vi "myRIO-1900 Customized FPGA.vi"() -> ()   [LabVIEW 2021]
doc: "This VI contains the default FPGA personality in addition to code that generates a sine waveform and filtered sine waveform based on parameters set by RT Main.vi. Keeping the default personality allows you to continue using the myRIO APIs even after adding custom FPGA code."
uses:
  <vilib>/eio/EIONode/EIONode.xnode
  <vilib>/rvi/eio/common/nirviEmuTemplateMethod_errors.vi
  <vilib>/Platform/TimedLoop/XDataNode/wakeup.ctl
  <vilib>/Platform/TimedLoop/XDataNode/XDNodeRunTimeDep.lvlib
  <vilib>/Platform/TimedLoop/XDataNode/nitl_modes.ctl
  <vilib>/Platform/TimedLoop/XDataNode/timing_clust.ctl
  <vilib>/Platform/TimedLoop/XDataNode/XDataNode.xnode
  <vilib>/rvi/Analysis/measure/notch/XNode/niFpgaNotchFilter.xnode
  <vilib>/rvi/DataTransferAndStorage/Container/XNode/niFpgaContainer.xnode
  <vilib>/rvi/interface/RandomDataEmulation/nirviRandomDataFpgaReadWriteTemplate.vi
  <vilib>/rvi/LocalResourceManager/LocalResourceManager.xnode
  <vilib>/rvi/eio/common/nirviEmuReportErrorAndStop.vi
  <vilib>/rvi/DataTransferAndStorage/Container/Common/niFpgaContainerGetUniqueNameForEmu.vi
  <vilib>/rvi/DataTransferAndStorage/Container/Common/niFpgaContainerSetEmuInfo.vi
  <vilib>/rvi/FIFO/Fifo_Resource/nirvififoEmulationRead.vi
  <vilib>/rvi/FIFO/Fifo_Resource/nirvififoEmulationWrite.vi
  Sub VIs/Utilities/Start Boolean.ctl
panel:
  in  "SPI.A.IRQ.NO":u8=15
  in  "SPI.B.IRQ.NO":u8=15
  out "ACC.Z.VAL 2":u16
  out "SYS.ACC.RDY":bool
  out "ACC.Y.VAL 2":u16
  out "ACC.X.VAL 2":u16
  in  "Stop":bool
  in  "Sine wave properties":T1={"Frequency (periods/tick)"=0.0002500000409781933, "Phase offset (periods)"=0.0, "Scale factor"=1.0, "Amplitude offset"=0.0}
  in  "Initialize":bool
  in  "Filter scaled coefficients":i32[](array[numeric])=[-917062152, 995401988, -1407710991]
  out "Actual loop rate":u32=1000
  in  "Desired loop rate (ticks)":u32=1000
  out "AO.SYS.STAT":bool
  out "DI.BTN":u8 format="%08b"
  in  "DO.LED3:0":u8 format="%04b"
  in  "AO.SYS.GO":T2
  in  "AO.AudioOut_L.VAL":u16
  in  "AO.AudioOut_R.VAL":u16
  out "AI.AudioIn_L.VAL":u16
  out "AI.AudioIn_R.VAL":u16
  in  "DIO.B_15:8.OUT":u8 format="%08b"
  in  "DIO.B_15:8.DIR":u8 format="%08b"
  out "DIO.B_15:8.IN":u8 format="%08b"
  in  "DIO.A_15:8.DIR":u8 format="%08b"
  in  "DIO.A_15:8.OUT":u8 format="%08b"
  out "DIO.A_15:8.IN":u8 format="%08b"
  in  "PWM.C_0.MAX":u16
  in  "PWM.C_0.CMP":u16
  out "PWM.C_0.CNTR":u16
  in  "PWM.C_0.CNFG":u8 format="%08b"
  in  "PWM.C_0.CS":u8
  in  "PWM.C_1.MAX":u16
  in  "PWM.C_1.CMP":u16
  out "PWM.C_1.CNTR":u16
  in  "PWM.C_1.CNFG":u8 format="%08b"
  in  "PWM.C_1.CS":u8
  out "ENC.C_1.STAT":u8 format="%08b"
  out "ENC.C_1.CNTR":u32
  in  "ENC.C_1.CNFG":u8 format="%08b"
  out "ENC.C_0.STAT":u8 format="%08b"
  out "ENC.C_0.CNTR":u32
  in  "ENC.C_0.CNFG":u8 format="%08b"
  in  "SYS.SELECTA":u8 format="%08b"
  in  "SYS.SELECTC":u8 format="%08b"
  in  "SYS.SELECTB":u8 format="%08b"
  in  "AO.C_1.VAL":u16
  in  "AO.C_0.VAL":u16
  out "AI.C_0.VAL":u16
  out "AI.C_1.VAL":u16
  in  "DIO.C_7:0.OUT":u8 format="%08b"
  in  "DIO.C_7:0.DIR":u8 format="%08b"
  out "DIO.C_7:0.IN":u8 format="%08b"
  in  "DIO.A_7:0.DIR":u8 format="%08b"
  in  "DIO.A_7:0.OUT":u8 format="%08b"
  out "DIO.A_7:0.IN":u8 format="%08b"
  in  "PWM.B_0.CMP":u16
  in  "PWM.B_0.MAX":u16
  out "PWM.B_0.CNTR":u16
  in  "PWM.B_0.CNFG":u8 format="%08b"
  in  "PWM.B_0.CS":u8
  in  "PWM.B_1.CMP":u16
  in  "PWM.B_1.MAX":u16
  out "PWM.B_1.CNTR":u16
  in  "PWM.B_1.CNFG":u8 format="%08b"
  in  "PWM.B_1.CS":u8
  in  "PWM.B_2.CMP":u16
  in  "PWM.B_2.MAX":u16
  out "PWM.B_2.CNTR":u16
  in  "PWM.B_2.CNFG":u8 format="%08b"
  in  "PWM.B_2.CS":u8
  out "SYS.RDY":bool
  out "SYS.AI.RDY":bool
  in  "I2C.B.GO":T2
  in  "I2C.A.GO":T2
  in  "I2C.A.CNFG":u8 format="%08b"
  in  "I2C.B.CNFG":u8 format="%08b"
  in  "I2C.A.DATO":u8
  out "I2C.A.DATI":u8
  in  "I2C.A.ADDR":u8 format="%08b"
  in  "I2C.A.CNTR":u8
  in  "I2C.B.DATO":u8
  out "I2C.B.DATI":u8
  in  "I2C.B.ADDR":u8 format="%08.0f"
  in  "I2C.B.CNTR":u8
  in  "I2C.A.CNTL":u8 format="%08b"
  out "I2C.A.STAT":u8 format="%08b"
  in  "I2C.B.CNTL":u8 format="%08b"
  out "I2C.B.STAT":u8 format="%08b"
  out "SPI.B.STAT":u8 format="%08b"
  in  "SPI.B.GO":T2
  out "SPI.A.STAT":u8 format="%08b"
  in  "SPI.A.GO":T2
  out "ENC.B.STAT":u8 format="%08b"
  out "ENC.A.STAT":u8 format="%08b"
  out "ENC.B.CNTR":u32
  out "ENC.A.CNTR":u32
  in  "ENC.B.CNFG":u8 format="%08b"
  in  "ENC.A.CNFG":u8 format="%08b"
  in  "SPI.B.DATO":u16
  out "SPI.B.DATI":u16
  in  "SPI.B.CNFG":u16 format="%016.0f"
  in  "SPI.B.CNT":u16
  in  "SPI.A.CNT":u16
  in  "SPI.A.CNFG":u16 format="%016b"
  out "SPI.A.DATI":u16
  in  "SPI.A.DATO":u16
  in  "PWM.A_0.MAX":u16
  in  "PWM.A_0.CMP":u16
  out "PWM.A_0.CNTR":u16
  in  "PWM.A_0.CNFG":u8 format="%08b"
  in  "PWM.A_0.CS":u8
  in  "PWM.A_1.CMP":u16
  in  "PWM.A_1.MAX":u16
  out "PWM.A_1.CNTR":u16
  in  "PWM.A_1.CNFG":u8 format="%08b"
  in  "PWM.A_1.CS":u8
  in  "PWM.A_2.CMP":u16
  in  "PWM.A_2.MAX":u16
  out "PWM.A_2.CNTR":u16
  in  "PWM.A_2.CNFG":u8 format="%08b"
  in  "PWM.A_2.CS":u8
  in  "DIO.B_7:0.OUT":u8 format="%08b"
  in  "DIO.B_7:0.DIR":u8 format="%08b"
  out "DIO.B_7:0.IN":u8 format="%08b"
  out "AI.A_0.VAL":u16
  out "AI.A_1.VAL":u16
  out "AI.A_2.VAL":u16
  out "AI.A_3.VAL":u16
  out "AI.B_0.VAL":u16
  out "AI.B_1.VAL":u16
  out "AI.B_2.VAL":u16
  out "AI.B_3.VAL":u16
  in  "AO.B_1.VAL":u16
  in  "AO.B_0.VAL":u16
  in  "AO.A_1.VAL":u16
  in  "AO.A_0.VAL":u16
  # "System"
  # "Onboard Devices"
  # "Connector A"
  # "Connector B"
  # "Connector C"
  # "Audio Connector"
  # "Accelerometer"
  # "Analog Input"
  # "Analog Output"
  # "Digital I/O"
  # "Counters / PWM"
  # "SPI Master"
  # "Analog Input"
  # "Analog Output"
  # "Digital I/O"
  # "Counters / PWM"
  # "SPI Master"
  # "Analog Input"
  # "Analog Output"
  # "Digital I/O"
  # "Counters / PWM"
  # "Analog Input"
  # "Analog Output"
  # "Encoders"
  # "IO Configuration"
  # "Buttons & LEDs"
  # "IO Configuration"
  # "IO Configuration"
  # "Encoders"
  # "Encoders"
  # "I2C Master"
  # "I2C Master"
  # "This VI contains the default FPGA personality in addition to code that generates a sine waveform and filtered sine waveform based on parameters set by RT Main.vi. Keeping the default personality allows you to continue using the myRIO APIs even after adding custom FPGA code."
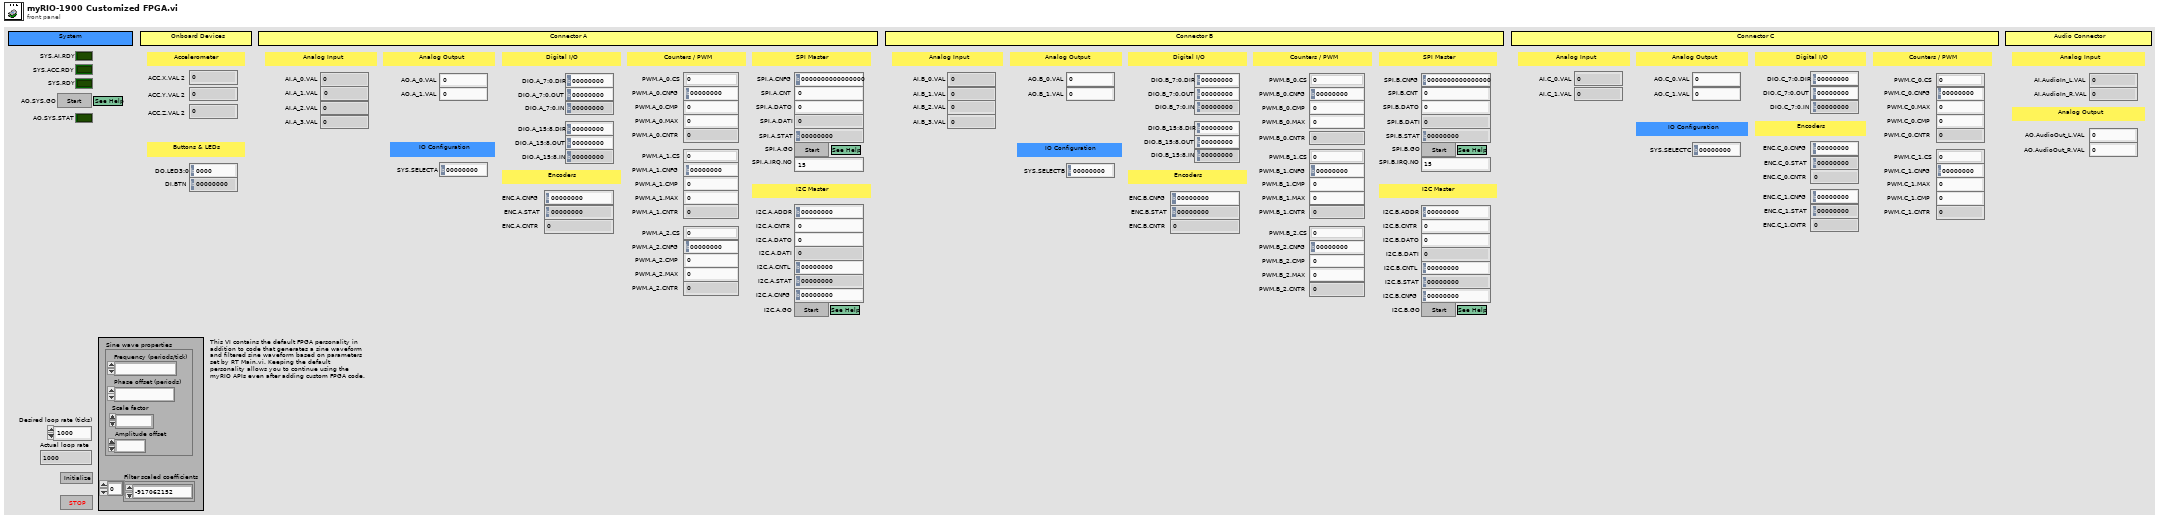
[diagram p1: front panel]
types:
  T1 = cluster{"Frequency (periods/tick)":fxp<+,32,0>, "Phase offset (periods)":fxp<+,32,0>, "Scale factor":fxp<+,12,1>, "Amplitude offset":fxp<+/-,16,12>}
  T2 = typedef "Start Boolean.ctl" = bool
  T3 = typedef "XDNodeRunTimeDep.lvlib/timing_clust.ctl" = cluster{"Expected End [f-1]":u64, "Actual End [f-1]":u64, "Finished Late? [f-1]":bool, "Expected End [i-1]":u64, "Actual End [i-1]":u64, "Finished Late? [i-1]":bool, "Expected Start [i]":u64, "Actual Start [i]":u64, "Expected Start [f]":u64, "Actual Start [f]":u64, "Source Name":string, "Structure Name":string, "Period":i64, "Deadline":i64, "Offset":i64, "Start":i64, "Priority":i32, "Timeout":i32, "Mode":T4, "Wakeup Reason":T5, "Error":errorcluster, "Source Type":string, "Secondary Source Type":string, "Global End Time":u64, "Global Start Time":u64, "Frame Duration":u64, "Iteration Duration":u64, "Assigned CPU":i32, "I/O Scan Engine Mode":u32}
  T4 = typedef "XDNodeRunTimeDep.lvlib/nitl_modes.ctl" = enum32{"No Change", "Process missed periods, maintain original phase", "Discard missed periods, maintain original phase", "Process missed periods, ignore original phase", "Discard missed periods, ignore original phase"}
  T5 = typedef "XDNodeRunTimeDep.lvlib/wakeup.ctl" = enum32{"Normal", "Aborted", "Asynchronous wakeup", "Timing source error", "Timed loop error", "Timeout"}
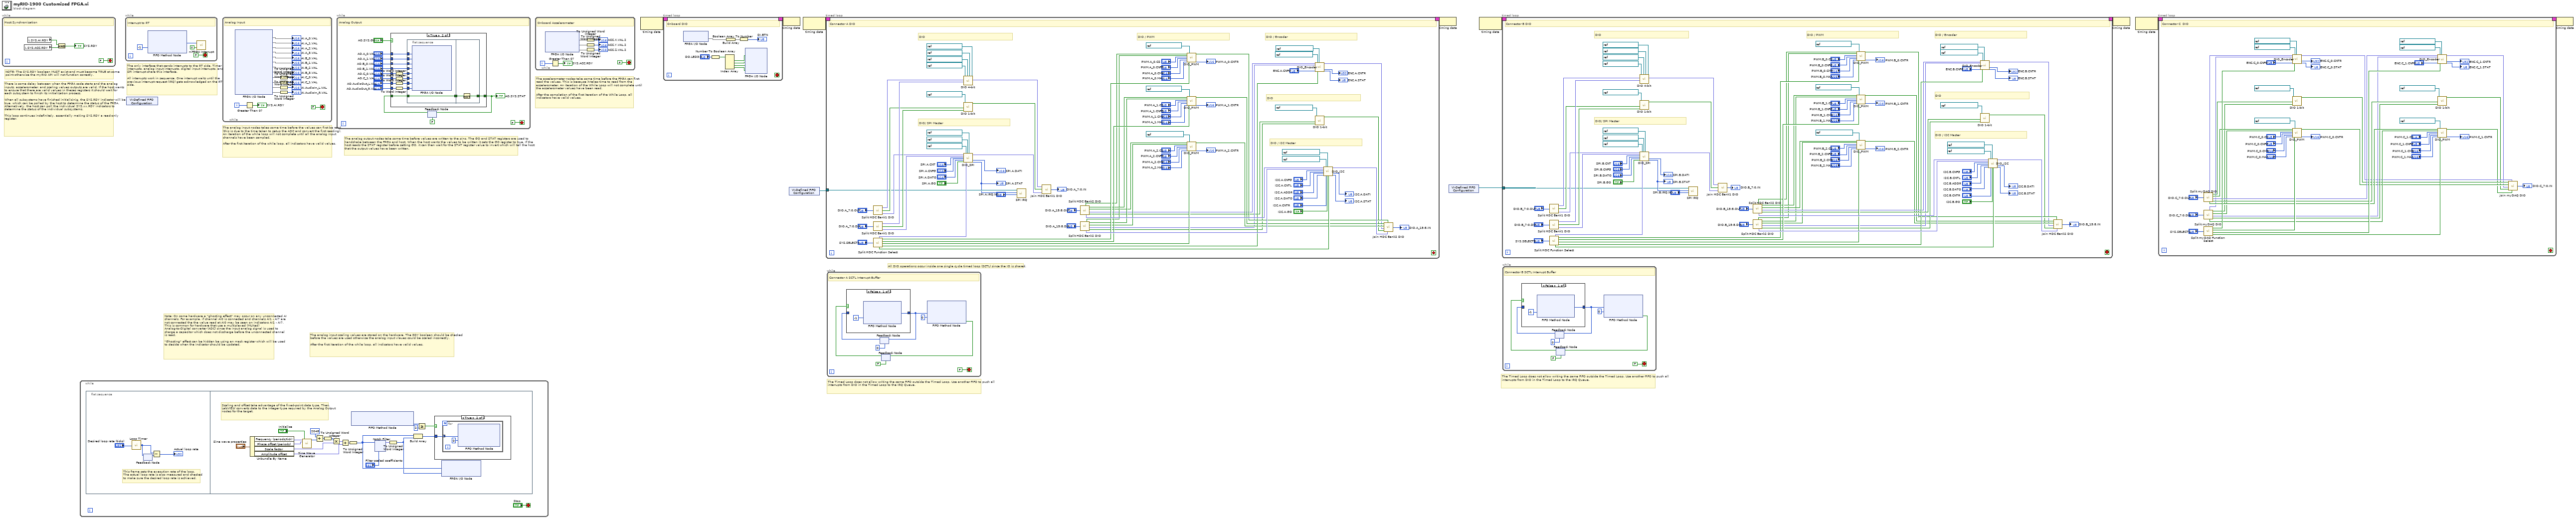
[diagram p0: block diagram]
diagram:
  # "The Timed Loop does not allow writing the same FIFO outside the Timed Loop. Use another FIFO to push all interrupts from DIO in the Timed Loop to the IRQ Queue."
  # "The Timed Loop does not allow writing the same FIFO outside the Timed Loop. Use another FIFO to push all interrupts from DIO in the Timed Loop to the IRQ Queue."
  # "The only interface that sends interrupts to the RT side. Timer interrupts, analog input interrupts, digital input interrupts, and SPI interrupt share this interface.\n\nAll interrupts work in sequence. One interrupt waits until the previous interrupt request (IRQ) gets acknowledged on the RT side."
  # "The accelerometer nodes take some time before the FPGA can first read the values. This is because it takes time to read from the accelerometer. An iteration of the While Loop will not complete until the accelerometer values have been read.\n\nAfter the completion of the first iteration of the While Loop, all indicators have valid values."
  # "NOTE: The SYS.RDY boolean MUST exist and must become TRUE at some point otherwise the myRIO API will not function correctly."
  # "All DIO operations occur inside one single cycle timed loop (SCTL) since the IO is shared."
  # "The analog input scaling values are stored on the hardware. The RDY boolean should be checked before the values are used otherwise the analog input vlaues could be scaled incorrectly.\n\nAfter the first iteration of the while loop, all indicators have valid values."
  # "There is some delay between when the FPGA code starts and the analog inputs, accelerometer, and scaling values outputs are valid. If the host wants to ensure that there are valid values in theses registers it should wait for each subsystem to finish its initialization process. \n\nWhen all subsystems have finished initializinig, the SYS.RDY indicator will be true, which can be polled by the host to determine the status of the FPGA. Alternatively, the host can poll the individual SYS.xx.RDY indicators to determine the status of the individual subsystems.\n\nThis loop continues indefinitely, essentially making SYS.RDY a read-only register."
  # "The analog input nodes takes some time before the values can first be read (this is due to the time taken to setup the ADC and convert the first reading). An iteration of the while loop will not complete until all the analog input channels have been sampled.\n\nAfter the first iteration of the while loop, all indicators have valid values."
  # "Note: On some hardware a \"ghosting effect\" may occur on any unconnected AI channels. For example, if channel AI0 is connected and channels AI1 - AI7 are not connected the the value read at AI0 may be seen on indicators AI1 - AI7. This is common for hardware that use a multiplexed (MUXed) Analog-to-Digital converter (ADC) since the input analog signal is used to charge a capacitor which does not discharge before the unconnected channel is read.\n\n\"Ghosting\" effect can be hidden be using an mask register which will be used to decide when the indicator should be updated."
  # "The analog output nodes take some time before values are written to the pins. The GO and STAT registers are used to handshake between the FPGA and host. When the host wants the values to be written it sets the GO register to true. If the host reads the STAT register before setting GO, it can then wait for the STAT register value to invert which will tell the host that the output values have been written."
  n1 = while {
    stop <- FALSE stop-if-true
    # "Host Synchronization"
    n2 = local read "SYS.ACC.RDY"() -> (w11:bool)
    n3 = local read "SYS.AI.RDY"() -> (w14:bool)
    n4 = Compound Arithmetic op=AND(w14, w11) -> (→"SYS.RDY":bool)
  }
  n5 = while {
    stop <- "Stop" stop-if-true
    n6 = flat-sequence {
      frame #0 {
        # "This frame sets the execution rate of the loop.\nThe actual loop rate is also measured and checked\nto make sure the desired loop rate is achieved."
        n7 = call "Loop Timer"("Count(Ticks)"="Desired loop rate (ticks)") -> ("Tick Count(Ticks)"=w17:u32)
        n8 = feedback-in #1(w17) -> ()
        n9 = feedback #1() -> (w18:u32)  [unwired: 1 out]
        n10 = Subtract(x=w17, y=w18) -> (x-y=→"Actual loop rate":u32)
      }
      frame #1 {
        # "Scaling and offset take advantage of the fixed-point data type. Then, LabVIEW converts data to the integer type required by the Analog Output nodes for the target."
        n11 = Unbundle By Name("Sine wave properties") -> ("Frequency (periods/tick)"=w36:fxp<+,32,0>, "Phase offset (periods)"=w35:fxp<+,32,0>, "Scale factor"=w38:fxp<+,12,1>, "Amplitude offset"=w37:fxp<+/-,16,12>)
        n12 = call "Sine Wave Generator"("frequency (periods/tick)"=w36, "reset"="Initialize", "phase offset (periods)"=w35) -> ("sine out"=w26:i16)  [unwired: 12 in]
        n13 = Add(x=i16 2048, y=w26) -> (x+y=w24:i16)
        n14 = To Unsigned Word Integer(number=w24) -> (unsigned 16bit integer=w23:u16)
        n15 = Multiply(x=w23, y=w38) -> (x*y=w34:fxp<+,28,17>)
        n16 = Add(x=w34, y=w37) -> (x+y=w33:fxp<+,12,12>)
        n17 = To Unsigned Word Integer(number=w33) -> (unsigned 16bit integer=w22:u16)
        n18 = xnode ("FIFO Method Node")() -> ("Number of Elements to Write"=w30:u32)  [unwired: 1 in, 1 out]
        n19 = xnode "Notch Filter"("input data"=w22, "scaled coefficients"="Filter scaled coefficients") -> ("output data"=w21:fxp<+/-,17,17>)  [unwired: 1 in]
        n20 = To Unsigned Word Integer(number=w21) -> (unsigned 16bit integer=w20:u16)
        n21 = Build Array(w22, w20) -> (w31:u16[])
        n22 = Greater Or Equal?(x=w30, y=u32 2) -> (x >= y?=w28:bool)
        n23 = case shown="True" w28 {
          tunnel: w31 -> [_ w40]
          frame False {
          }
          frame True {
            n24 = for {
              tunnel: w40 -> [w41] mode=indexing
              n25 = xnode ("FIFO Method Node")("Element"=w41, "Timeout"=0) -> ()  [unwired: 1 in, 2 out]
            }
          }
        }
        n26 = xnode "FPGA I/O Node"("ConnectorA/AO0"=w22, "ConnectorA/AO1"=w20) -> ()  [unwired: 2 in, 2 out]
      }
    }
  }
  n27 = while {
    stop <- FALSE stop-if-true
    # "Interrupt to RT"
    n28 = xnode ("FIFO Method Node")("Timeout"=-1) -> ("Element"=w51:u8)  [unwired: 1 in, 2 out]
    n29 = call <vilib>:"niFPGA Interrupt.vi"("Wait Until Cleared (F)"=TRUE, "IRQ Number (0)"=w51) -> ()  [unwired: 1 in]
  }
  n30 = xnode "VI-Defined FIFO Configuration"() -> ()  [unwired: 1 out]
  n31 = while {
    i -> [w68]
    stop <- FALSE stop-if-true
    # "Analog Input"
    n32 = xnode "FPGA I/O Node"() -> ("ConnectorA/AI0"=→"AI.A_0.VAL", "ConnectorA/AI1"=→"AI.A_1.VAL", "ConnectorA/AI2"=→"AI.A_2.VAL", "ConnectorA/AI3"=→"AI.A_3.VAL", "ConnectorB/AI0"=→"AI.B_0.VAL", "ConnectorB/AI1"=→"AI.B_1.VAL", "ConnectorB/AI2"=→"AI.B_2.VAL", "ConnectorB/AI3"=→"AI.B_3.VAL", "ConnectorC/AI0"=w62, "ConnectorC/AI1"=w61, "AudioIn/Left"=w60, "AudioIn/Right"=w59)  [unwired: 12 in, 12 out]
    n33 = Greater Than 0?(x=w68) -> (x > 0?=→"SYS.AI.RDY":bool)
    n34 = To Unsigned Word Integer(number=w62) -> (unsigned 16bit integer=→"AI.C_0.VAL":u16)
    n35 = To Unsigned Word Integer(number=w61) -> (unsigned 16bit integer=→"AI.C_1.VAL":u16)
    n36 = To Unsigned Word Integer(number=w60) -> (unsigned 16bit integer=→"AI.AudioIn_L.VAL":u16)
    n37 = To Unsigned Word Integer(number=w59) -> (unsigned 16bit integer=→"AI.AudioIn_R.VAL":u16)
  }
  n38 = while {
    stop <- FALSE stop-if-true
    # "Analog Output"
    n39 = feedback #2(FALSE) -> (w76:bool)
    n40 = case shown="True" "AO.SYS.GO" {
      tunnel: "AO.C_0.VAL" -> [_ w98]
      tunnel: "AO.C_1.VAL" -> [_ w97]
      tunnel: "AO.A_0.VAL" -> [_ w102]
      tunnel: "AO.A_1.VAL" -> [_ w101]
      tunnel: "AO.B_0.VAL" -> [_ w100]
      tunnel: "AO.B_1.VAL" -> [_ w99]
      tunnel: "AO.AudioOut_L.VAL" -> [_ w94]
      tunnel: "AO.AudioOut_R.VAL" -> [_ w93]
      tunnel: w76 -> [w87 w90]
      tunnel: [w87 w88] -> w74
      frame False {
      }
      frame True {
        n41 = To Word Integer(number=w98) -> (16bit integer=w96:i16)
        n42 = To Word Integer(number=w97) -> (16bit integer=w95:i16)
        n43 = To Word Integer(number=w94) -> (16bit integer=w92:i16)
        n44 = To Word Integer(number=w93) -> (16bit integer=w91:i16)
        n45 = flat-sequence {
          tunnel: w102 -> [w111]
          tunnel: w101 -> [w110]
          tunnel: w100 -> [w109]
          tunnel: w99 -> [w108]
          tunnel: w96 -> [w107]
          tunnel: w95 -> [w106]
          tunnel: w92 -> [w105]
          tunnel: w91 -> [w104]
          tunnel: w90 -> [w103]
          tunnel: [w103] -> w89
          tunnel: w89 -> [w113]
          tunnel: [w112] -> w88
          frame #0 {
            n46 = xnode "FPGA I/O Node"("ConnectorA/AO0"=w111, "ConnectorA/AO1"=w110, "ConnectorB/AO0"=w109, "ConnectorB/AO1"=w108, "ConnectorC/AO0"=w107, "ConnectorC/AO1"=w106, "AudioOut/Left"=w105, "AudioOut/Right"=w104) -> ()  [unwired: 8 in, 8 out]
          }
          frame #1 {
            n47 = Not(x=w113) -> (.not. x?=w112:bool)
          }
        }
      }
    }
    "AO.SYS.STAT" <- w74
    n48 = feedback-in #2(w74) -> ()
  }
  n49 = while {
    i -> [w118]
    stop <- FALSE stop-if-true
    # "Onboard Accelerometer"
    n50 = xnode "FPGA I/O Node"() -> ("AccelerationX"=w121, "AccelerationY"=w120, "AccelerationZ"=w119)  [unwired: 3 in, 3 out]
    n51 = Greater Than 0?(x=w118) -> (x > 0?=→"SYS.ACC.RDY":bool)
    n52 = To Unsigned Word Integer(number=w121) -> (unsigned 16bit integer=→"ACC.X.VAL 2":u16)
    n53 = To Unsigned Word Integer(number=w120) -> (unsigned 16bit integer=→"ACC.Y.VAL 2":u16)
    n54 = To Unsigned Word Integer(number=w119) -> (unsigned 16bit integer=→"ACC.Z.VAL 2":u16)
  }
  n55 = node-c288() -> (w4:T3)  [unwired: 1 in]
  n56 = timed-loop {
    timing: w4 -> [_]
    timing-out: [_] -> w3
    stop <- _ stop-if-true
    # "Onboard DIO"
    n57 = xnode "FPGA I/O Node"() -> ("Button0"=w123)  [unwired: 1 in, 1 out]
    n58 = Number To Boolean Array(number="DO.LED3:0") -> (Boolean array=w128:bool[])
    n59 = Index Array(array=w128) -> (element #1=w127:bool, element #2=w126:bool, element #3=w125:bool, element #4=w124:bool)  [unwired: 4 in]
    n60 = Build Array(w123) -> (w131:void[])
    n61 = Boolean Array To Number(Boolean array=w131) -> (number=→"DI.BTN":u8)
    n62 = xnode "FPGA I/O Node"("LED0"=w127, "LED1"=w126, "LED2"=w125, "LED3"=w124) -> ()  [unwired: 4 in, 4 out]
  }
  n63 = node-c288(w3) -> ()
  n64 = xnode "VI-Defined FIFO Configuration"() -> ("FIFO Out"=w1:refnum<k21>)
  n65 = node-c288() -> (w8:T3)  [unwired: 1 in]
  n66 = timed-loop {
    timing: w8 -> [_]
    timing-out: [_] -> w7
    tunnel: w1 -> [w136]
    stop <- _ stop-if-true
    # "DIO / Encoder"
    # "DIO / I2C Master"
    # "DIO / PWM"
    # "DIO"
    # "DIO"
    # "DIO/ SPI Master"
    # "Connector A DIO"
    n67 = call "Split HDC Bank1 DIO.vi"("IN 7:0"="DIO.A_7:0.OUT") -> ("OUT 3:0"=w223:fxp<+,4,4>, "OUT 4"=w138:bool, "OUT 7:5"=w220:fxp<+,3,3>)
    n68 = call "Split HDC Bank1 DIO.vi"("IN 7:0"="DIO.A_7:0.DIR") -> ("OUT 3:0"=w222:fxp<+,4,4>, "OUT 4"=w221:bool, "OUT 7:5"=w219:fxp<+,3,3>)
    n69 = call "Split HDC Function Select.vi"("IN 7:0"="SYS.SELECTA") -> ("OUT 1:0"=w159:fxp<+,2,2>, "OUT 7"=w154:bool, "OUT 2"=w158:bool, "OUT 3"=w157:bool, "OUT 4"=w156:bool, "OUT 5"=w155:bool)
    n70 = call "DIO 4-bit.vi"("DIO0 Refnum"=refnum<k21> "ConnectorA/DIO0", "DIO1 Refnum"=refnum<k21> "ConnectorA/DIO1", "DIO2 Refnum"=refnum<k21> "ConnectorA/DIO2", "DIR 3:0"=w222, "OUT 3:0"=w223, "DIO3 Refnum"=refnum<k21> "ConnectorA/DIO3") -> ("IN 3:0"=w137:fxp<+,4,4>)  [unwired: 5 in]
    n71 = call "DIO 1-bit.vi"("DIR"=w221, "OUT"=w138, "DIO Refnum"=refnum<k21> "ConnectorA/DIO4") -> ("IN"=w195:bool)  [unwired: 8 in]
    n72 = call "DIO_SPI.vi"("DIO.2:0.OUT"=w220, "DIO.2:0.DIR"=w219, "SPI.CNT"="SPI.A.CNT", "SPI.CNFG"="SPI.A.CNFG", "SPI.DATO"="SPI.A.DATO", "SPI.GO"="SPI.A.GO", "DIO.2/SPI.MOSI Refnum"=refnum<k21> "ConnectorA/DIO7" ("DIO.2/SPI.SCLK"), "SELECT.1:0"=w159, "DIO.1/SPI.MISO Refnum"=refnum<k21> "ConnectorA/DIO6" ("DIO.1/SPI.MOSI"), "DIO.0/SPI.SCLK Refnum"=refnum<k21> "ConnectorA/DIO5" ("DIO.0/SPI.MISO")) -> ("DIO.2:0.IN"=w194:fxp<+,3,3>, "SPI.DATI"=→"SPI.A.DATI":u16, "SPI.STAT"=w135:u8)  [unwired: 7 in]
    "SPI.A.STAT" <- w135
    n73 = call "SPI IRQ.vi"("SPI.A.IRQ.NO"="SPI.A.IRQ.NO", "SPI.STAT"=w135, "FIFO In"=w136) -> ()  [unwired: 9 in]
    n74 = call "Join HDC Bank1 DIO.vi"("IN 7:5"=w194, "IN 4"=w195, "IN 3:0"=w137) -> ("OUT 7:0"=→"DIO.A_7:0.IN":u8)
    n75 = call "Split HDC Bank2 DIO.vi"("IN 7:0"="DIO.A_15:8.OUT") -> ("OUT 5"=w140:bool, "OUT 7:6"=w164:fxp<+,2,2>, "OUT 4:3"=w142:fxp<+,2,2>, "OUT 2"=w144:bool, "OUT 0"=w148:bool, "OUT 1"=w147:bool)  [unwired: 2 in]
    n76 = call "Split HDC Bank2 DIO.vi"("IN 7:0"="DIO.A_15:8.DIR") -> ("OUT 5"=w139:bool, "OUT 7:6"=w163:fxp<+,2,2>, "OUT 4:3"=w141:fxp<+,2,2>, "OUT 2"=w143:bool, "OUT 0"=w146:bool, "OUT 1"=w145:bool)  [unwired: 2 in]
    n77 = call "DIO_PWM.vi"("DIO.OUT"=w148, "DIO.DIR"=w146, "PWM.CS"="PWM.A_0.CS", "PWM.CNFG"="PWM.A_0.CNFG", "PWM.CMP"="PWM.A_0.CMP", "PWM.MAX"="PWM.A_0.MAX", "DIO/PWM"=refnum<k21> "ConnectorA/DIO8", "SELECT"=w158) -> ("DIO.IN"=w153:bool, "PWM.CNTR"=→"PWM.A_0.CNTR":u16)  [unwired: 10 in]
    n78 = call "DIO_PWM.vi"("DIO.OUT"=w147, "DIO.DIR"=w145, "PWM.CS"="PWM.A_1.CS", "PWM.CNFG"="PWM.A_1.CNFG", "PWM.CMP"="PWM.A_1.CMP", "PWM.MAX"="PWM.A_1.MAX", "DIO/PWM"=refnum<k21> "ConnectorA/DIO9", "SELECT"=w157) -> ("DIO.IN"=w152:bool, "PWM.CNTR"=→"PWM.A_1.CNTR":u16)  [unwired: 10 in]
    n79 = call "DIO_PWM.vi"("DIO.OUT"=w144, "DIO.DIR"=w143, "PWM.CS"="PWM.A_2.CS", "PWM.CNFG"="PWM.A_2.CNFG", "PWM.CMP"="PWM.A_2.CMP", "PWM.MAX"="PWM.A_2.MAX", "DIO/PWM"=refnum<k21> "ConnectorA/DIO10", "SELECT"=w156) -> ("DIO.IN"=w151:bool, "PWM.CNTR"=→"PWM.A_2.CNTR":u16)  [unwired: 10 in]
    n80 = call "DIO_Encoder.vi"("DIO.1:0.OUT"=w142, "DIO.1:0.DIR"=w141, "QE.CNFG"="ENC.A.CNFG", "DIO.1/QE.B"=refnum<k21> "ConnectorA/DIO12", "SELECT"=w155, "DIO.0/QE.A"=refnum<k21> "ConnectorA/DIO11") -> ("DIO.1:0.IN"=w150:fxp<+,2,2>, "QE.CNTR"=→"ENC.A.CNTR":u32, "QE.STAT"=→"ENC.A.STAT":u8)  [unwired: 11 in]
    n81 = call "DIO 1-bit.vi"("DIR"=w139, "OUT"=w140, "DIO Refnum"=refnum<k21> "ConnectorA/DIO13") -> ("IN"=w149:bool)  [unwired: 8 in]
    n82 = call "DIO_I2C.vi"("DIO.1:0.OUT"=w164, "DIO.1:0.DIR"=w163, "I2C.CNFG"="I2C.A.CNFG", "I2C.CNTL"="I2C.A.CNTL", "I2C.ADDR"="I2C.A.ADDR", "I2C.DATO"="I2C.A.DATO", "DIO.1/I2C.SDA"=refnum<k21> "ConnectorA/DIO15" ("DIO.1/I2C.SCL"), "I2C.CNTR"="I2C.A.CNTR", "DIO.0/I2C.SCL"=refnum<k21> "ConnectorA/DIO14" ("DIO.0/I2C.SDA"), "Execute?"="I2C.A.GO", "SELECT"=w154) -> ("DIO.1:0.IN"=w161:fxp<+,2,2>, "I2C.DATI"=→"I2C.A.DATI":u8, "I2C.STAT"=→"I2C.A.STAT":u8)  [unwired: 6 in]
    n83 = call "Join HDC Bank2 DIO.vi"("IN 7:6"=w161, "IN 5"=w149, "IN 4:3"=w150, "IN 0"=w153, "IN 2"=w151, "IN 1"=w152) -> ("OUT 7:0"=→"DIO.A_15:8.IN":u8)  [unwired: 4 in]
  }
  n84 = while {
    stop <- FALSE stop-if-true
    # "Connector A SCTL Interrupt Buffer"
    n85 = feedback #3(u8 0 ("Element")) -> (w228:u8)
    n86 = feedback #4(FALSE ("Timed Out?")) -> (w232:bool)
    n87 = case shown="False" w232 {
      tunnel: [w234 w236] -> w229
      tunnel: w228 -> [_ w236]
      frame False {
        n88 = xnode ("FIFO Method Node")("Timeout"=-1) -> ("Element"=w234:u8)  [unwired: 1 in, 2 out]
      }
      frame True {
      }
    }
    n89 = feedback-in #3(w229) -> ()
    n90 = xnode ("FIFO Method Node")("Element"=w229, "Timeout"=0) -> ("Timed Out?"=w230:bool)  [unwired: 1 in, 1 out]
    n91 = feedback-in #4(w230) -> ()
  }
  n92 = node-c288(w7) -> ()
  n93 = xnode "VI-Defined FIFO Configuration"() -> ("FIFO Out"=w2:refnum<k21>)
  n94 = node-c288() -> (w6:T3)  [unwired: 1 in]
  n95 = timed-loop {
    timing: w6 -> [_]
    timing-out: [_] -> w5
    tunnel: w2 -> [w238]
    stop <- _ stop-if-true
    # "DIO / Encoder"
    # "DIO / I2C Master"
    # "DIO / PWM"
    # "DIO"
    # "DIO"
    # "DIO/ SPI Master"
    # "Connector B DIO"
    n96 = call "Split HDC Bank1 DIO.vi"("IN 7:0"="DIO.B_7:0.OUT") -> ("OUT 3:0"=w326:fxp<+,4,4>, "OUT 4"=w324:bool, "OUT 7:5"=w322:fxp<+,3,3>)
    n97 = call "Split HDC Bank1 DIO.vi"("IN 7:0"="DIO.B_7:0.DIR") -> ("OUT 3:0"=w325:fxp<+,4,4>, "OUT 4"=w323:bool, "OUT 7:5"=w321:fxp<+,3,3>)
    n98 = call "Split HDC Function Select.vi"("IN 7:0"="SYS.SELECTB") -> ("OUT 1:0"=w298:fxp<+,2,2>, "OUT 7"=w293:bool, "OUT 2"=w297:bool, "OUT 3"=w296:bool, "OUT 4"=w295:bool, "OUT 5"=w294:bool)
    n99 = call "DIO 4-bit.vi"("DIO0 Refnum"=refnum<k21> "ConnectorB/DIO0", "DIO1 Refnum"=refnum<k21> "ConnectorB/DIO1", "DIO2 Refnum"=refnum<k21> "ConnectorB/DIO2", "DIR 3:0"=w325, "OUT 3:0"=w326, "DIO3 Refnum"=refnum<k21> "ConnectorB/DIO3") -> ("IN 3:0"=w304:fxp<+,4,4>)  [unwired: 5 in]
    n100 = call "DIO 1-bit.vi"("DIR"=w323, "OUT"=w324, "DIO Refnum"=refnum<k21> "ConnectorB/DIO4") -> ("IN"=w303:bool)  [unwired: 8 in]
    n101 = call "DIO_SPI.vi"("DIO.2:0.OUT"=w322, "DIO.2:0.DIR"=w321, "SPI.CNT"="SPI.B.CNT", "SPI.CNFG"="SPI.B.CNFG", "SPI.DATO"="SPI.B.DATO", "SPI.GO"="SPI.B.GO", "DIO.2/SPI.MOSI Refnum"=refnum<k21> "ConnectorB/DIO7" ("DIO.2/SPI.SCLK"), "SELECT.1:0"=w298, "DIO.1/SPI.MISO Refnum"=refnum<k21> "ConnectorB/DIO6" ("DIO.1/SPI.MOSI"), "DIO.0/SPI.SCLK Refnum"=refnum<k21> "ConnectorB/DIO5" ("DIO.0/SPI.MISO")) -> ("DIO.2:0.IN"=w302:fxp<+,3,3>, "SPI.DATI"=→"SPI.B.DATI":u16, "SPI.STAT"=w239:u8)  [unwired: 7 in]
    "SPI.B.STAT" <- w239
    n102 = call "SPI IRQ.vi"("SPI.A.IRQ.NO"="SPI.B.IRQ.NO", "SPI.STAT"=w239, "FIFO In"=w238) -> ()  [unwired: 9 in]
    n103 = call "Join HDC Bank1 DIO.vi"("IN 7:5"=w302, "IN 4"=w303, "IN 3:0"=w304) -> ("OUT 7:0"=→"DIO.B_7:0.IN":u8)
    n104 = call "Split HDC Bank2 DIO.vi"("IN 7:0"="DIO.B_15:8.OUT") -> ("OUT 5"=w250:bool, "OUT 7:6"=w301:fxp<+,2,2>, "OUT 4:3"=w251:fxp<+,2,2>, "OUT 2"=w252:bool, "OUT 0"=w254:bool, "OUT 1"=w253:bool)  [unwired: 2 in]
    n105 = call "Split HDC Bank2 DIO.vi"("IN 7:0"="DIO.B_15:8.DIR") -> ("OUT 5"=w245:bool, "OUT 7:6"=w300:fxp<+,2,2>, "OUT 4:3"=w246:fxp<+,2,2>, "OUT 2"=w247:bool, "OUT 0"=w249:bool, "OUT 1"=w248:bool)  [unwired: 2 in]
    n106 = call "DIO_PWM.vi"("DIO.OUT"=w254, "DIO.DIR"=w249, "PWM.CS"="PWM.B_0.CS", "PWM.CNFG"="PWM.B_0.CNFG", "PWM.CMP"="PWM.B_0.CMP", "PWM.MAX"="PWM.B_0.MAX", "DIO/PWM"=refnum<k21> "ConnectorB/DIO8", "SELECT"=w297) -> ("DIO.IN"=w244:bool, "PWM.CNTR"=→"PWM.B_0.CNTR":u16)  [unwired: 10 in]
    n107 = call "DIO_PWM.vi"("DIO.OUT"=w253, "DIO.DIR"=w248, "PWM.CS"="PWM.B_1.CS", "PWM.CNFG"="PWM.B_1.CNFG", "PWM.CMP"="PWM.B_1.CMP", "PWM.MAX"="PWM.B_1.MAX", "DIO/PWM"=refnum<k21> "ConnectorB/DIO9", "SELECT"=w296) -> ("DIO.IN"=w243:bool, "PWM.CNTR"=→"PWM.B_1.CNTR":u16)  [unwired: 10 in]
    n108 = call "DIO_PWM.vi"("DIO.OUT"=w252, "DIO.DIR"=w247, "PWM.CS"="PWM.B_2.CS", "PWM.CNFG"="PWM.B_2.CNFG", "PWM.CMP"="PWM.B_2.CMP", "PWM.MAX"="PWM.B_2.MAX", "DIO/PWM"=refnum<k21> "ConnectorB/DIO10", "SELECT"=w295) -> ("DIO.IN"=w242:bool, "PWM.CNTR"=→"PWM.B_2.CNTR":u16)  [unwired: 10 in]
    n109 = call "DIO_Encoder.vi"("DIO.1:0.OUT"=w251, "DIO.1:0.DIR"=w246, "QE.CNFG"="ENC.B.CNFG", "DIO.1/QE.B"=refnum<k21> "ConnectorB/DIO12", "SELECT"=w294, "DIO.0/QE.A"=refnum<k21> "ConnectorB/DIO11") -> ("DIO.1:0.IN"=w241:fxp<+,2,2>, "QE.CNTR"=→"ENC.B.CNTR":u32, "QE.STAT"=→"ENC.B.STAT":u8)  [unwired: 11 in]
    n110 = call "DIO 1-bit.vi"("DIR"=w245, "OUT"=w250, "DIO Refnum"=refnum<k21> "ConnectorB/DIO13") -> ("IN"=w240:bool)  [unwired: 8 in]
    n111 = call "DIO_I2C.vi"("DIO.1:0.OUT"=w301, "DIO.1:0.DIR"=w300, "I2C.CNFG"="I2C.B.CNFG", "I2C.CNTL"="I2C.B.CNTL", "I2C.ADDR"="I2C.B.ADDR", "I2C.DATO"="I2C.B.DATO", "DIO.1/I2C.SDA"=refnum<k21> "ConnectorB/DIO15" ("DIO.1/I2C.SCL"), "I2C.CNTR"="I2C.B.CNTR", "DIO.0/I2C.SCL"=refnum<k21> "ConnectorB/DIO14" ("DIO.0/I2C.SDA"), "Execute?"="I2C.B.GO", "SELECT"=w293) -> ("DIO.1:0.IN"=w299:fxp<+,2,2>, "I2C.DATI"=→"I2C.B.DATI":u8, "I2C.STAT"=→"I2C.B.STAT":u8)  [unwired: 6 in]
    n112 = call "Join HDC Bank2 DIO.vi"("IN 7:6"=w299, "IN 5"=w240, "IN 4:3"=w241, "IN 0"=w244, "IN 2"=w242, "IN 1"=w243) -> ("OUT 7:0"=→"DIO.B_15:8.IN":u8)  [unwired: 4 in]
  }
  n113 = while {
    stop <- FALSE stop-if-true
    # "Connector B SCTL Interrupt Buffer"
    n114 = feedback #5(u8 0 ("Element")) -> (w333:u8)
    n115 = feedback #6(FALSE ("Timed Out?")) -> (w335:bool)
    n116 = case shown="False" w335 {
      tunnel: [w337 w339] -> w330
      tunnel: w333 -> [_ w339]
      frame False {
        n117 = xnode ("FIFO Method Node")("Timeout"=-1) -> ("Element"=w337:u8)  [unwired: 1 in, 2 out]
      }
      frame True {
      }
    }
    n118 = feedback-in #5(w330) -> ()
    n119 = xnode ("FIFO Method Node")("Element"=w330, "Timeout"=0) -> ("Timed Out?"=w329:bool)  [unwired: 1 in, 1 out]
    n120 = feedback-in #6(w329) -> ()
  }
  n121 = node-c288(w5) -> ()
  n122 = node-c288() -> (w10:T3)  [unwired: 1 in]
  n123 = timed-loop {
    timing: w10 -> [_]
    timing-out: [_] -> w9
    stop <- _ stop-if-true
    # "Connector C  DIO"
    n124 = call "Split myDAQ DIO.vi"("IN 7:0"="DIO.C_7:0.OUT") -> ("OUT 2, OUT0"=w358:fxp<+,2,2>, "OUT 1"=w357:bool, "OUT 3"=w356:bool, "OUT 7"=w353:bool, "OUT 6, OUT 4"=w355:fxp<+,2,2>, "OUT 5"=w354:bool)  [unwired: 4 in]
    n125 = call "Split myDAQ DIO.vi"("IN 7:0"="DIO.C_7:0.DIR") -> ("OUT 2, OUT0"=w352:fxp<+,2,2>, "OUT 1"=w351:bool, "OUT 3"=w350:bool, "OUT 7"=w347:bool, "OUT 6, OUT 4"=w349:fxp<+,2,2>, "OUT 5"=w348:bool)  [unwired: 4 in]
    n126 = call "Split myDAQ Function Select.vi"("IN 7:0"="SYS.SELECTC") -> ("OUT 0"=w364:bool, "OUT 1"=w363:bool, "OUT 2"=w362:bool, "OUT 3"=w361:bool)  [unwired: 2 in]
    n127 = call "DIO_Encoder.vi"("DIO.1:0.OUT"=w358, "DIO.1:0.DIR"=w352, "QE.CNFG"="ENC.C_0.CNFG", "DIO.1/QE.B"=refnum<k21> "ConnectorC/DIO2", "SELECT"=w364, "DIO.0/QE.A"=refnum<k21> "ConnectorC/DIO0") -> ("DIO.1:0.IN"=w345:fxp<+,2,2>, "QE.CNTR"=→"ENC.C_0.CNTR":u32, "QE.STAT"=→"ENC.C_0.STAT":u8)  [unwired: 11 in]
    n128 = call "DIO 1-bit.vi"("DIR"=w351, "OUT"=w357, "DIO Refnum"=refnum<k21> "ConnectorC/DIO1") -> ("IN"=w344:bool)  [unwired: 8 in]
    n129 = call "DIO_PWM.vi"("DIO.OUT"=w356, "DIO.DIR"=w350, "PWM.CS"="PWM.C_0.CS", "PWM.CNFG"="PWM.C_0.CNFG", "PWM.CMP"="PWM.C_0.CMP", "PWM.MAX"="PWM.C_0.MAX", "DIO/PWM"=refnum<k21> "ConnectorC/DIO3", "SELECT"=w363) -> ("DIO.IN"=w343:bool, "PWM.CNTR"=→"PWM.C_0.CNTR":u16)  [unwired: 10 in]
    n130 = call "DIO_Encoder.vi"("DIO.1:0.OUT"=w355, "DIO.1:0.DIR"=w349, "QE.CNFG"="ENC.C_1.CNFG", "DIO.1/QE.B"=refnum<k21> "ConnectorC/DIO6", "SELECT"=w362, "DIO.0/QE.A"=refnum<k21> "ConnectorC/DIO4") -> ("DIO.1:0.IN"=w342:fxp<+,2,2>, "QE.CNTR"=→"ENC.C_1.CNTR":u32, "QE.STAT"=→"ENC.C_1.STAT":u8)  [unwired: 11 in]
    n131 = call "DIO 1-bit.vi"("DIR"=w348, "OUT"=w354, "DIO Refnum"=refnum<k21> "ConnectorC/DIO5") -> ("IN"=w341:bool)  [unwired: 8 in]
    n132 = call "DIO_PWM.vi"("DIO.OUT"=w353, "DIO.DIR"=w347, "PWM.CS"="PWM.C_1.CS", "PWM.CNFG"="PWM.C_1.CNFG", "PWM.CMP"="PWM.C_1.CMP", "PWM.MAX"="PWM.C_1.MAX", "DIO/PWM"=refnum<k21> "ConnectorC/DIO7", "SELECT"=w361) -> ("DIO.IN"=w340:bool, "PWM.CNTR"=→"PWM.C_1.CNTR":u16)  [unwired: 10 in]
    n133 = call "Join myDAQ DIO.vi"("IN 7"=w340, "IN 5"=w341, "IN 6, IN 4"=w342, "IN 2, IN 0"=w345, "IN 3"=w343, "IN 1"=w344) -> ("IN 7:0"=→"DIO.C_7:0.IN":u8)  [unwired: 4 in]
  }
  n134 = node-c288(w9) -> ()
